vi "Destroy.vi"(8 "error in (no error)":errorcluster, 11 "Plugin Manager in":refnum<class "CIFPluginManager.lvclass">) -> (0 "error out":errorcluster, 3 "Plugin Manager out":refnum<class "CIFPluginManager.lvclass">)   [LabVIEW 2021, in "CIFPluginManager.lvclass"]
uses:
  CIFPluginManager.lvclass
  <vilib>/CIF Foundation/CIF Core/CIFUtilities/CIFLogs/Typedef/Message Type.ctl
  typedef/Loader Map.ctl
  typedef/Loaders.ctl
  typedef/Loader Type.ctl
  <vilib>/gRPC/LabVIEW gRPC Library/Shared/grpcId.ctl
  typedef/Plugin Management Data Map.ctl
  typedef/Plugin Management Data.ctl
  <vilib>/CIF Foundation/CIF Core/CIFCore/Common/Typedef/Version.ctl
  gRPC/CIF_Manager_server/RPC Messages/cif_management_common_PluginStatusData.ctl
  gRPC/CIF_Manager_server/RPC Messages/cif_management_common_PluginStatusData_PluginState.ctl
  gRPC/CIF_Manager_server/RPC Messages/cif_management_common_TimingStatistics.ctl
  gRPC/CIF_Manager_server/RPC Messages/cif_common_TimingStats.ctl
  gRPC/CIF_Manager_server/RPC Messages/cif_management_common_FifoStatistics.ctl
  gRPC/CIF_Manager_server/RPC Messages/cif_management_common_Error.ctl
  gRPC/CIF_Manager_server/RPC Messages/cif_management_common_MonitorDoubles.ctl
  gRPC/CIF_Manager_server/RPC Messages/cif_management_common_MonitorU64.ctl
  gRPC/CIF_Manager_server/RPC Messages/cif_management_common_MonitorI64.ctl
  gRPC/CIF_Manager_server/RPC Messages/cif_management_common_Channels.ctl
  gRPC/CIF_Manager_server/RPC Messages/cif_management_common_Channel.ctl
  gRPC/CIF_Manager_server/RPC Messages/cif_management_common_ChannelDirection.ctl
  gRPC/CIF_Manager_server/RPC Messages/cif_management_common_ChannelPattern.ctl
  CIFPluginManager.lvclass/CIFPluginManager.ctl
  <vilib>/gRPC/LabVIEW gRPC Library/Client API/Close Client.vi
  <vilib>/gRPC/LabVIEW gRPC Servicer/ServiceBase/ServiceBase.lvclass
  <vilib>/CIF Foundation/CIF Core/CIFUtilities/CIFLogs/CIFLogs.lvlib
  <vilib>/gRPC/LabVIEW gRPC Library/grpc-lvsupport-release.lvlib
  <vilib>/CIF Foundation/CIF Core/CIFCore/Common/CIFCoreCommon.lvlib
  gRPC/CIF_Manager_server/CIF_Manager_server.lvlib
  <vilib>/gRPC/LabVIEW gRPC Servicer/Servicer/Servicer.lvclass
  <vilib>/CIF Foundation/CIF Core/CIFCore/Grpc/CIFCoreWrapper/CIFCoreWrapper.lvlib
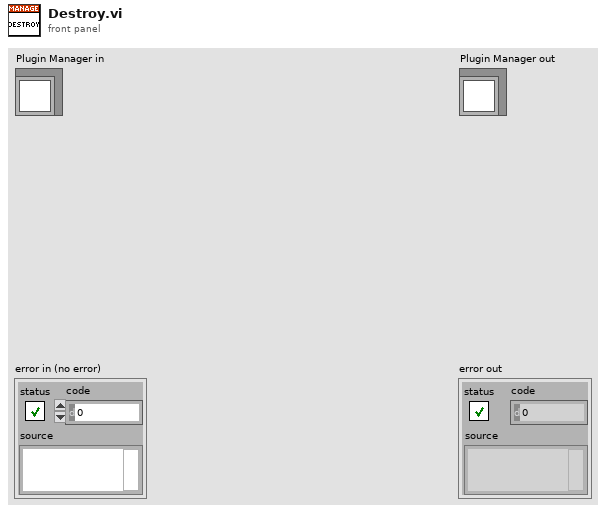
[diagram p1: front panel]
types:
  T1 = typedef "CIFLogs.lvlib/Message Type.ctl" = enum16{"Error", "Information", "Print Terminal", "Configuration"}
  T2 = typedef "CIFPluginManager.lvclass/Plugin Management Data Map.ctl" = map{string, T3}
  T3 = typedef "CIFPluginManager.lvclass/Plugin Management Data.ctl" = cluster{"Unique Name":string, "Plugin Type":string, "gRPC Port":i32, "gRPC ID":T4, "Loader Type":T5, "Loader":string, "Version":T6, "Load Timestamp":i64, "Unload Timestamp":i64, "Unloading":bool, "Ready for removal":bool, "status":T7, "channels":T16}
  T4 = typedef "grpc-lvsupport-release.lvlib/grpcId.ctl" = u64
  T5 = typedef "CIFPluginManager.lvclass/Loader Type.ctl" = enum16{"LabVIEW"}
  T6 = typedef "CIFCoreCommon.lvlib/Version.ctl" = cluster{"Major":i32, "Minor":i32, "Fix":i32, "Build":i32}
  T7 = typedef "CIF_Manager_server.lvlib/cif_management_common_PluginStatusData.ctl" = cluster{"state":T8, "timing_statistics":T9, "fifo_statistics":T11, "error":T12, "monitor_doubles":T13, "monitor_u64s":T14, "monitor_i64s":T15}
  T8 = typedef "CIF_Manager_server.lvlib/cif_management_common_PluginStatusData_PluginState.ctl" = enum32{"PLUGINSTATE_UNKNOWN", "PLUGINSTATE_CREATING", "PLUGINSTATE_LISTENING", "PLUGINSTATE_RUNNING", "PLUGINSTATE_CLEANINGUP", "PLUGINSTATE_DESTROYING"}
  T9 = typedef "CIF_Manager_server.lvlib/cif_management_common_TimingStatistics.ctl" = cluster{"period":T10, "wake_error":T10, "execute":T10, "housekeep":T10, "idle":T10, "cleanup":T10, "custom_1":T10, "custom_2":T10}
  T10 = typedef "CIF_Manager_server.lvlib/cif_common_TimingStats.ctl" = cluster{"max":i64, "min":i64, "avg":dbl}
  T11 = typedef "CIF_Manager_server.lvlib/cif_management_common_FifoStatistics.ctl" = cluster{"from_t0":T10, "from_previous_plugin":T10, "output_error":T10}
  T12 = typedef "CIF_Manager_server.lvlib/cif_management_common_Error.ctl" = cluster{"status":bool, "code":i32}
  T13 = typedef "CIF_Manager_server.lvlib/cif_management_common_MonitorDoubles.ctl" = cluster{"double_1":dbl, "double_2":dbl, "double_3":dbl, "double_4":dbl}
  T14 = typedef "CIF_Manager_server.lvlib/cif_management_common_MonitorU64.ctl" = cluster{"u64_1":u64, "u64_2":u64, "u64_3":u64, "u64_4":u64}
  T15 = typedef "CIF_Manager_server.lvlib/cif_management_common_MonitorI64.ctl" = cluster{"i64_1":i64, "i64_2":i64, "i64_3":i64, "i64_4":i64}
  T16 = typedef "CIF_Manager_server.lvlib/cif_management_common_Channels.ctl" = cluster{"channels":T17[]}
  T17 = typedef "CIF_Manager_server.lvlib/cif_management_common_Channel.ctl" = cluster{"name":string, "direction":T18, "type":string, "custom_config":u8[], "connected":bool, "connected_name":string, "forced":bool, "channel_pattern":T19}
  T18 = typedef "CIF_Manager_server.lvlib/cif_management_common_ChannelDirection.ctl" = enum32{"CHANNELDIRECTION_UNKNOWN", "CHANNELDIRECTION_PUBLISHER", "CHANNELDIRECTION_SUBSCRIBER"}
  T19 = typedef "CIF_Manager_server.lvlib/cif_management_common_ChannelPattern.ctl" = enum32{"CHANNELPATTERN_UNKNOWN", "CHANNELPATTERN_TAG", "CHANNELPATTERN_FIFO", "CHANNELPATTERN_MULTIFIFO", "CHANNELPATTERN_BACKPRESSUREFIFO"}
  T20 = typedef "CIFPluginManager.lvclass/Loader Map.ctl" = map{string, T21}
  T21 = typedef "CIFPluginManager.lvclass/Loaders.ctl" = cluster{"Loader Type":T5, "grpc_port":i32, "pid":u32, "gRPC ID":T4, "Load Timestamp":i64, "Unloading":bool, "Ready for removal":bool, "Unload Timestamp":i64}
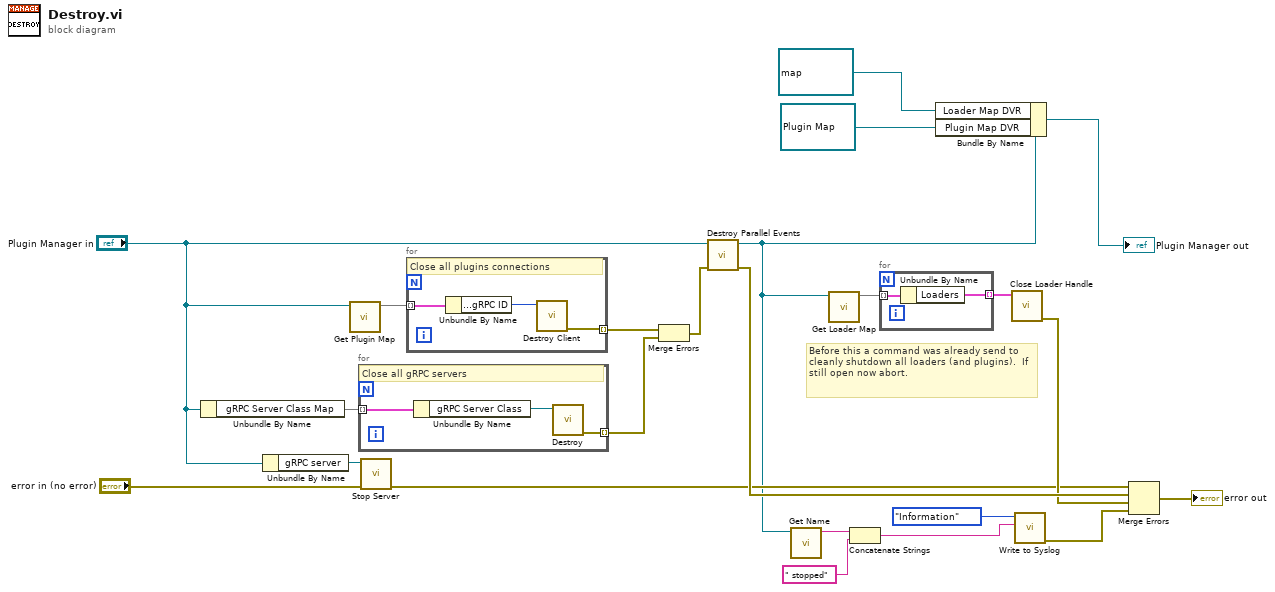
[diagram p0: block diagram]
diagram:
  # "Before this a command was already send to cleanly shutdown all loaders (and plugins).  If still open now abort."
  n1 = Unbundle By Name("Plugin Manager in") -> ("gRPC Server Class Map"=w1:map{string, refnum<class "ServiceBase.lvclass">})
  n2 = Unbundle By Name("Plugin Manager in") -> ("gRPC server"=w6:refnum<class "Servicer.lvclass">)
  n3 = call "Get Plugin Map.vi"("CIFPluginManager in"="Plugin Manager in") -> ("Plugin Map"=w17:T2)  [unwired: 9 in, 1 out]
  n4 = for {
    tunnel: w1 -> [w26] mode=indexing
    tunnel: [w24] -> w16 mode=indexing
    # "Close all gRPC servers"
    n5 = Unbundle By Name(w26) -> ("gRPC Server Class"=w25:refnum<class "ServiceBase.lvclass">)
    n6 = call-dynamic "Destroy.vi"("gRPC service in"=w25) -> ("error out"=w24:errorcluster)  [unwired: 9 in, 1 out]
  }
  n7 = call <vilib>:"Stop Server.vi"("error in"="error in (no error)", "gRPC server in"=w6) -> ("error out"=w7:errorcluster)  [unwired: 9 in]
  n8 = for {
    tunnel: w17 -> [w29] mode=indexing
    tunnel: [w27] -> w19 mode=indexing
    # "Close all plugins connections"
    n9 = Unbundle By Name(w29) -> ("Plugin Management Data.gRPC ID"=w28:T4)
    n10 = call <vilib>:"Destroy Client.vi"("gRPC ID"=w28) -> ("error out"=w27:errorcluster)  [unwired: 10 in]
  }
  n11 = Merge Errors(w19, w16) -> (w13:errorcluster)
  n12 = call "Destroy Parallel Events.vi"("error in (no error)"=w13, "CIFPluginManager in"="Plugin Manager in") -> ("error out"=w21:errorcluster, "CIFPluginManager out"=w2:refnum<class "CIFPluginManager.lvclass">)  [unwired: 8 in]
  n13 = call "Get Name.vi"("CIFPluginManager in"=w2) -> ("Name"=w5:string)  [unwired: 10 in]
  n14 = call "Get Loader Map.vi"("CIFPluginManager in"=w2) -> ("Loader Map"=w20:T20)  [unwired: 9 in, 1 out]
  n15 = Concatenate Strings(w5, " stopped" ("message")) -> (w3:string)
  n16 = for {
    tunnel: w20 -> [w31] mode=indexing
    tunnel: [w30] -> w11 mode=indexing
    n17 = Unbundle By Name(w31) -> ("Loaders"=w30:T21)
  }
  n18 = Bundle By Name(cluster=w2, "Loader Map DVR"=refnum<data-value> refnum, "Plugin Map DVR"=refnum<data-value> refnum) -> (→"Plugin Manager out":refnum<class "CIFPluginManager.lvclass">)
  n19 = call "Close Loader Handle.vi"("Loaders"=w11) -> ("error out"=w10:errorcluster)  [unwired: 10 in]
  n20 = call <vilib>:"Write to Syslog.vi"("message"=w3, "CIF Message Type"=Message_Type."Information") -> ("error out"=w12:errorcluster)  [unwired: 9 in]
  n21 = Merge Errors(w7, w21, w10, w12) -> (→"error out":errorcluster)
